vi "OCV Check for Faults.vi"(8 "Error In":errorcluster caption="error in", 10 "dmm voltage measurements":dbl[](array[numeric])) -> (0 "Error Out":errorcluster caption="error out", 1 "Voltage Out":dbl format="%#_6p", 2 "DMM Fault":bool)   [LabVIEW 2019]
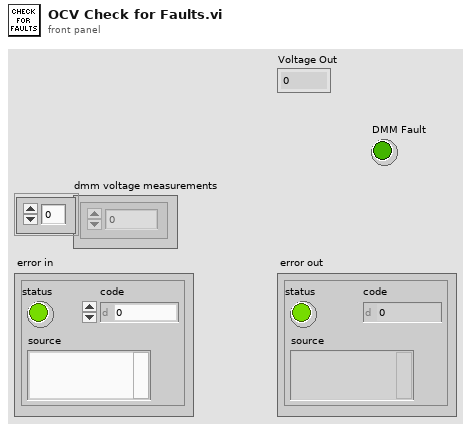
[diagram p1: front panel]
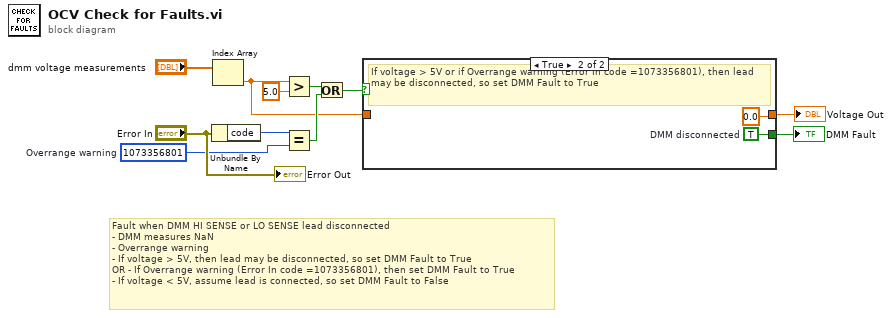
[diagram p0: block diagram]
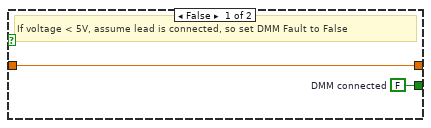
[diagram p2: hidden frame]
diagram:
  w8 = 1073356801  # Overrange warning
  # "Fault when DMM HI SENSE or LO SENSE lead disconnected\n- DMM measures NaN\n- Overrange warning\n- If voltage > 5V, then lead may be disconnected, so set DMM Fault to True\nOR - If Overrange warning (Error In code =1073356801), then set DMM Fault to True \n- If voltage < 5V, assume lead is connected, so set DMM Fault to False"
  n1 = Unbundle By Name("Error In") -> ("code"=w9:i32)
  n2 = Index Array(array="dmm voltage measurements") -> (element=w1:dbl)  [unwired: 1 in]
  n3 = Greater?(x=w1, y=5.0) -> (0:w7:bool)
  n4 = Equal?(x=w9, y=w8) -> (x = y?=w6:bool)
  n5 = Or(x=w7, y=w6) -> (x .or. y?=w5:bool)
  n6 = case shown="True" w5 {
    tunnel: [w13 w15] -> w4
    tunnel: [w12 0.0 ("Resistance In")] -> w2
    tunnel: w1 -> [w12 _]
    frame False {
      w13 = FALSE  # DMM connected
      # "If voltage < 5V, assume lead is connected, so set DMM Fault to False"
    }
    frame True {
      w15 = TRUE  # DMM disconnected
      # "If voltage > 5V or if Overrange warning (Error In code =1073356801), then lead may be disconnected, so set DMM Fault to True"
    }
  }
  "DMM Fault" <- w4
  "Voltage Out" <- w2
  "Error Out" <- "Error In"
